vi "Sub_Online_FEA.vi"(8 "Bound Search":bool, 9 "Mode Count":i32=3 min=1 max=10 step=1, 10 "Eigenvalue Method":T2(ring), 11 "Experiment In":T1) -> (3 "Experiment Out":T1)   [LabVIEW 2021]
uses:
  <vilib>/Analysis/7linalg.llb/Eigenvalue and Vectors Output Option.ctl
  <vilib>/Analysis/baseanly.llb/Matrix Type of Inverse Matrix.ctl
  <vilib>/Analysis/7linalg.llb/Real Generalized Eigenvalues and Vectors.vi
  <vilib>/Analysis/7linalg.llb/Real Cholesky Factorization.vi
  <vilib>/Analysis/baseanly.llb/Full Cholesky Factorization.vi
  <vilib>/Analysis/baseanly.llb/Full Real Matrix Cholesky Factorization.vi
  <vilib>/Analysis/Matrix/Numeric/Conversions/Array To Matrix - RA2.vi
  <vilib>/Analysis/baseanly.llb/Real Inverse Matrix.vi
  <vilib>/Analysis/Matrix/Numeric/Multiply/Multiply - RM,RM.vi
  <vilib>/Analysis/7linalg.llb/Real Eigenvalues and Vectors.vi
  <vilib>/Analysis/Matrix/Numeric/Add/Add - RM,RM.vi
  <vilib>/Analysis/NI_AALPro.lvlib
  <vilib>/Analysis/Matrix/NI_Matrix.lvlib
  <vilib>/Analysis/NI_AALBase.lvlib
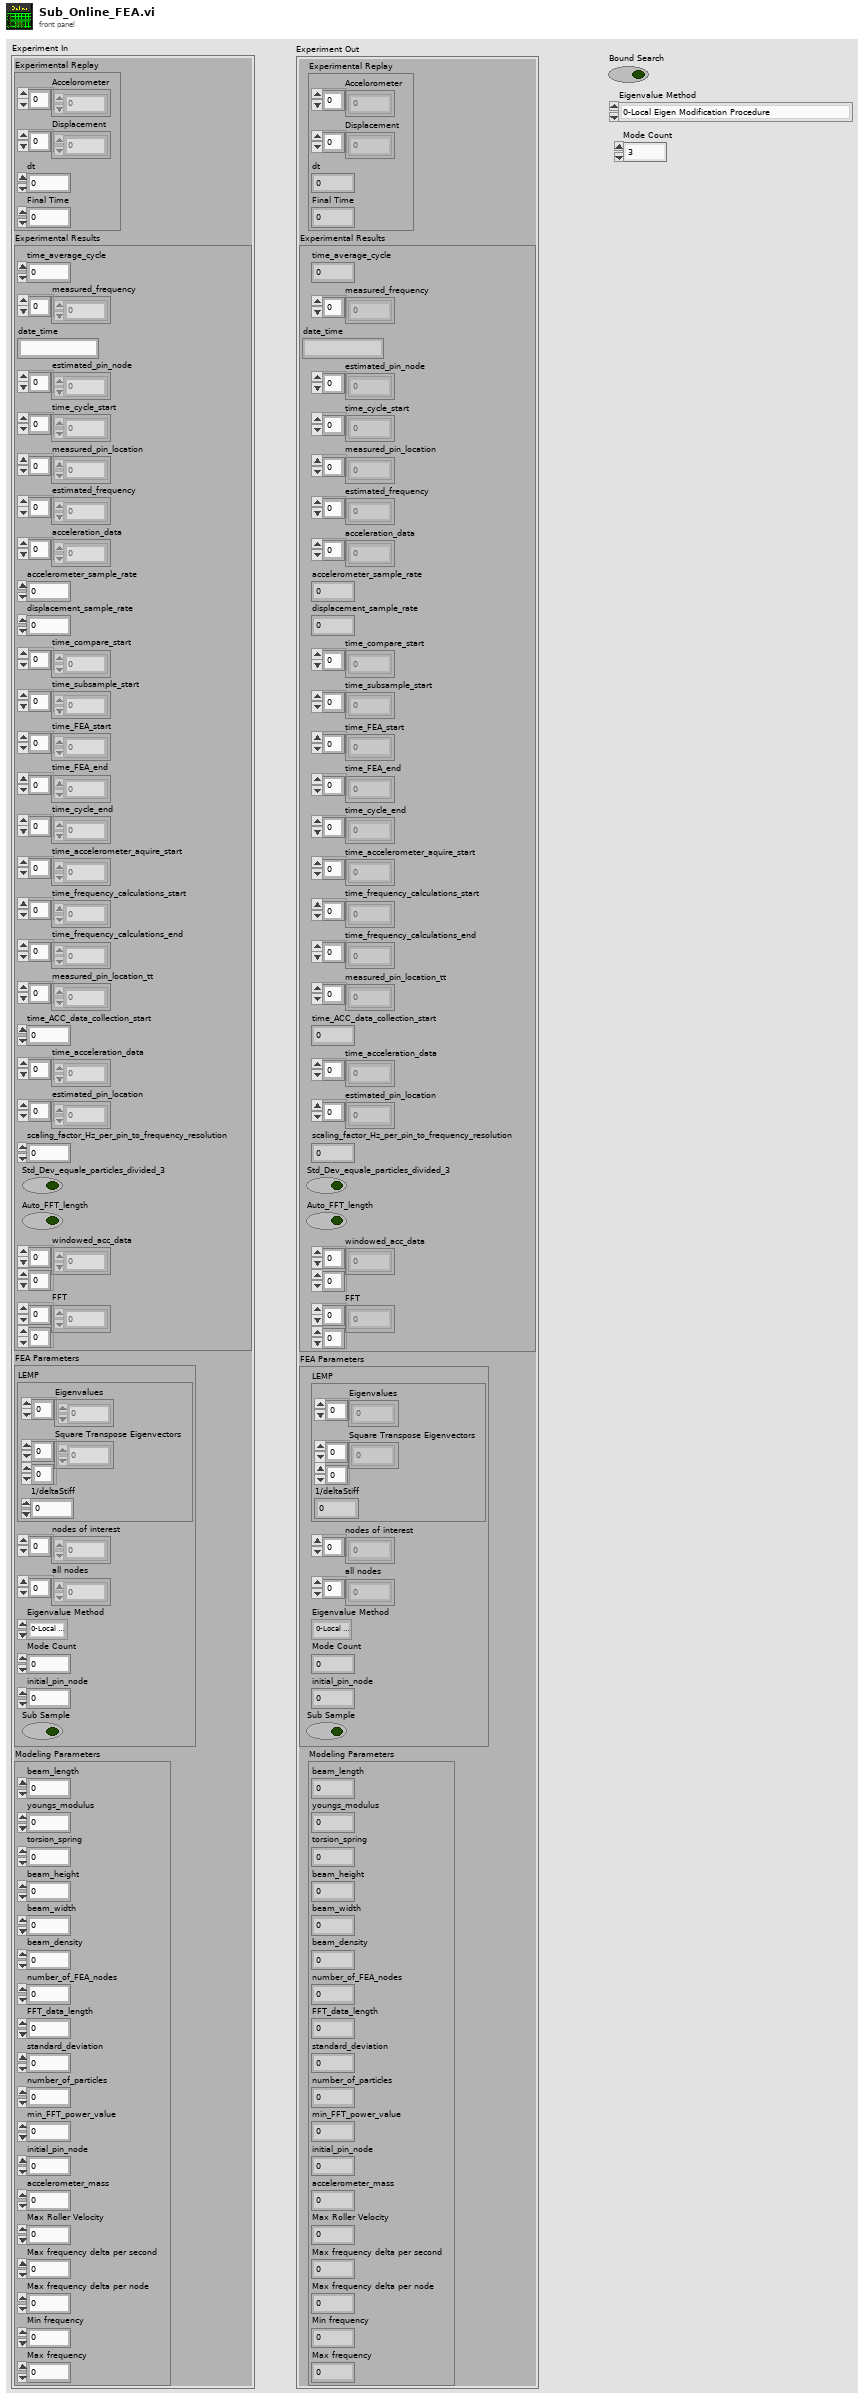
[diagram p1: front panel]
types:
  T1 = cluster{"Experimental Replay":cluster{"Accelorometer":dbl[], "Displacement":dbl[], "dt":dbl, "Final Time":dbl}, "Experimental Results":cluster{"time_average_cycle":dbl, "measured_frequency":dbl[], "date_time":string, "estimated_pin_node":i32[], "time_cycle_start":dbl[], "measured_pin_location":dbl[], "estimated_frequency":dbl[], "acceleration_data":dbl[], "accelerometer_sample_rate":dbl, "displacement_sample_rate":dbl, "time_compare_start":dbl[], "time_subsample_start":dbl[], "time_FEA_start":dbl[], "time_FEA_end":dbl[], "time_cycle_end":dbl[], "time_accelerometer_aquire_start":dbl[], "time_frequency_calculations_start":dbl[], "time_frequency_calculations_end":dbl[], "measured_pin_location_tt":dbl[], "time_ACC_data_collection_start":dbl, "time_acceleration_data":dbl[], "estimated_pin_location":dbl[], "scaling_factor_Hz_per_pin_to_frequency_resolution":dbl, "Std_Dev_equale_particles_divided_3":bool, "Auto_FFT_length":bool, "windowed_acc_data":dbl[][], "FFT":dbl[][]}, "FEA Parameters":cluster{"LEMP":cluster{"Eigenvalues":dbl[], "Square Transpose Eigenvectors":dbl[][], "1/deltaStiff":dbl}, "nodes of interest":i32[], "all nodes":i32[], "Eigenvalue Method":enum16{"0-Local Eigen Modification Procedure", "1-LabVIEW generalized eigenvalues", "2-LabVIEW M^-1K eigenvalues", "3-LabVIEW Cholesky Factorization", "4-Cholesky Factorization CPU SGL", "5-Cholesky Factorization CPU FXP", "6-Cholesky Factorization FPGA SGL", "7-Cholesky Factorization FPGA SGL SCL"}, "Mode Count":i32, "initial_pin_node":i32, "Sub Sample":bool}, "Modeling Parameters":cluster{"beam_length":dbl, "youngs_modulus":dbl, "torsion_spring":dbl, "beam_height":dbl, "beam_width":dbl, "beam_density":dbl, "number_of_FEA_nodes":i32, "FFT_data_length":i32, "standard_deviation":dbl, "number_of_particles":i32, "min_FFT_power_value":dbl, "initial_pin_node":i32, "accelerometer_mass":dbl, "Max Roller Velocity":dbl, "Max frequency delta per second":dbl, "Max frequency delta per node":dbl, "Min frequency":dbl, "Max frequency":dbl}}
  T2 = enum16{"0-Local Eigen Modification Procedure", "1-LabVIEW generalized eigenvalues", "2-LabVIEW M^-1K eigenvalues", "3-LabVIEW Cholesky Factorization", "4-Cholesky Factorization CPU SGL", "5-Cholesky Factorization CPU FXP", "6-Cholesky Factorization FPGA SGL", "7-Cholesky Factorization FPGA SGL SCL"}
  T3 = cluster{"LEMP":cluster{"Eigenvalues":dbl[], "Square Transpose Eigenvectors":dbl[][], "1/deltaStiff":dbl}, "nodes of interest":i32[], "all nodes":i32[], "Eigenvalue Method":enum16{"0-Local Eigen Modification Procedure", "1-LabVIEW generalized eigenvalues", "2-LabVIEW M^-1K eigenvalues", "3-LabVIEW Cholesky Factorization", "4-Cholesky Factorization CPU SGL", "5-Cholesky Factorization CPU FXP", "6-Cholesky Factorization FPGA SGL", "7-Cholesky Factorization FPGA SGL SCL"}, "Mode Count":i32, "initial_pin_node":i32, "Sub Sample":bool}
  T4 = cluster{"beam_length":dbl, "youngs_modulus":dbl, "torsion_spring":dbl, "beam_height":dbl, "beam_width":dbl, "beam_density":dbl, "number_of_FEA_nodes":i32, "FFT_data_length":i32, "standard_deviation":dbl, "number_of_particles":i32, "min_FFT_power_value":dbl, "initial_pin_node":i32, "accelerometer_mass":dbl, "Max Roller Velocity":dbl, "Max frequency delta per second":dbl, "Max frequency delta per node":dbl, "Min frequency":dbl, "Max frequency":dbl}
  T5 = cluster{"time_average_cycle":dbl, "measured_frequency":dbl[], "date_time":string, "estimated_pin_node":i32[], "time_cycle_start":dbl[], "measured_pin_location":dbl[], "estimated_frequency":dbl[], "acceleration_data":dbl[], "accelerometer_sample_rate":dbl, "displacement_sample_rate":dbl, "time_compare_start":dbl[], "time_subsample_start":dbl[], "time_FEA_start":dbl[], "time_FEA_end":dbl[], "time_cycle_end":dbl[], "time_accelerometer_aquire_start":dbl[], "time_frequency_calculations_start":dbl[], "time_frequency_calculations_end":dbl[], "measured_pin_location_tt":dbl[], "time_ACC_data_collection_start":dbl, "time_acceleration_data":dbl[], "estimated_pin_location":dbl[], "scaling_factor_Hz_per_pin_to_frequency_resolution":dbl, "Std_Dev_equale_particles_divided_3":bool, "Auto_FFT_length":bool, "windowed_acc_data":dbl[][], "FFT":dbl[][]}
  T6 = cluster{"Eigenvalues":dbl[], "Square Transpose Eigenvectors":dbl[][], "1/deltaStiff":dbl}
  T7 = typedef "NI_AALBase.lvlib/Matrix Type of Inverse Matrix.ctl" = enum32{"General", "Positive Definite", "Lower Triangular", "Upper Triangular"}
  T8 = typedef "NI_AALPro.lvlib/Eigenvalue and Vectors Output Option.ctl" = i32
  T9 = typedef "NI_Matrix.lvlib/RealMatrix.ctl" = dbl[][]
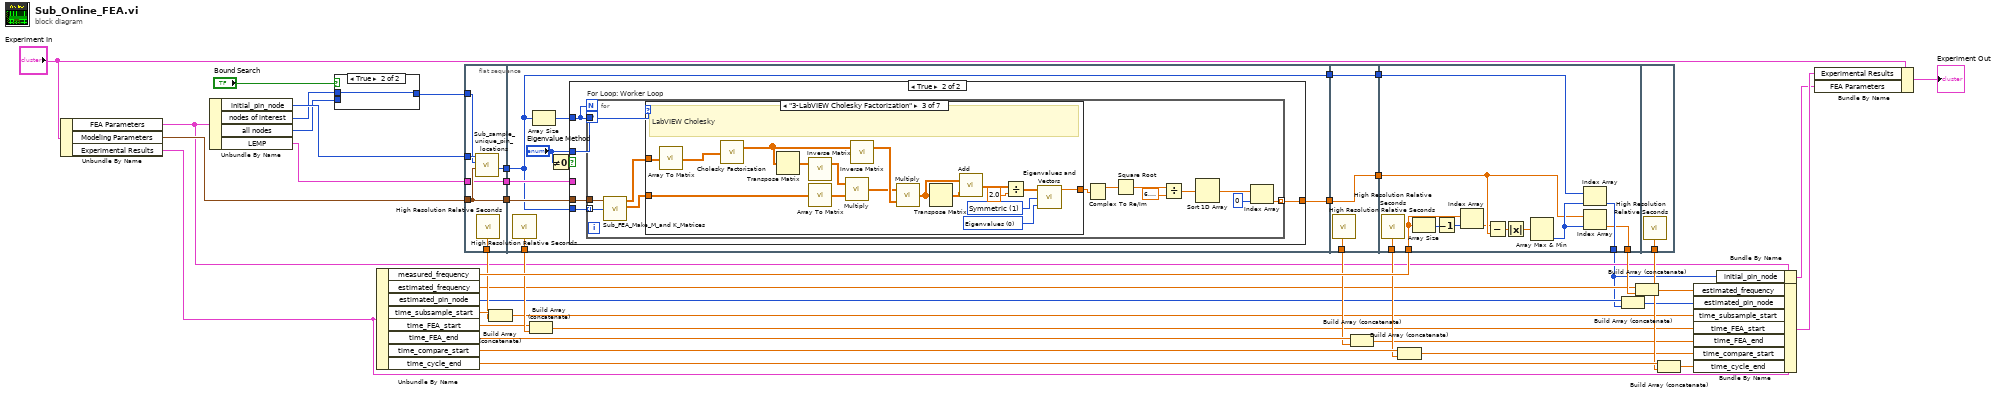
[diagram p0: block diagram]
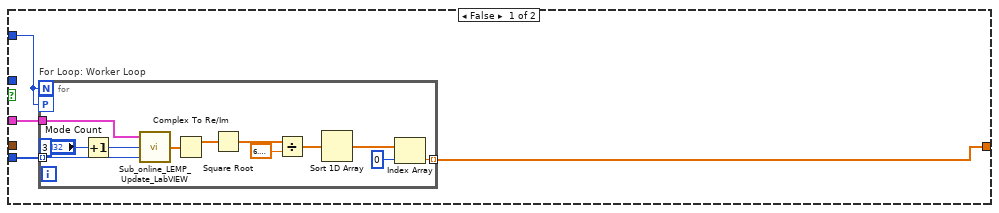
[diagram p3: hidden frame]
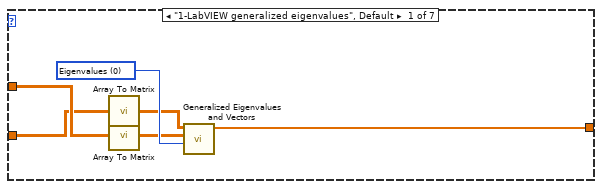
[diagram p4: hidden frame]
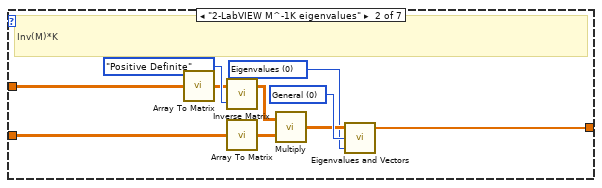
[diagram p5: hidden frame]
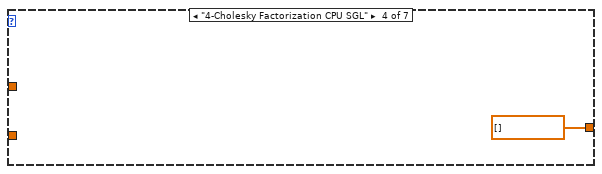
[diagram p6: hidden frame]
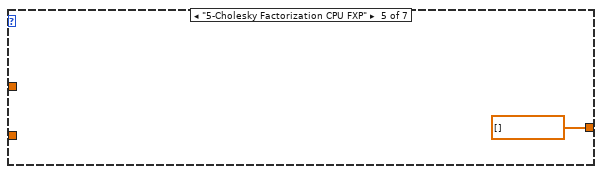
[diagram p7: hidden frame]
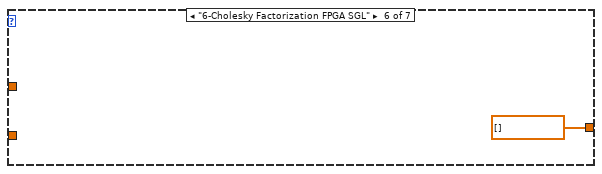
[diagram p8: hidden frame]
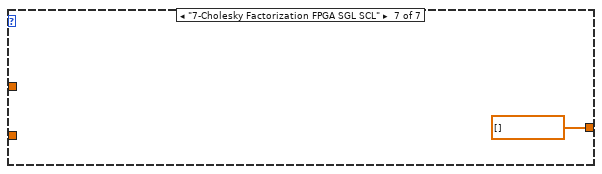
[diagram p9: hidden frame]
diagram:
  n1 = Unbundle By Name("Experiment In") -> ("FEA Parameters"=w3:T3, "Modeling Parameters"=w35:T4, "Experimental Results"=w14:T5)
  n2 = Unbundle By Name(w3) -> ("initial_pin_node"=w36:i32, "nodes of interest"=w34:i32[], "all nodes"=w33:i32[], "LEMP"=w32:T6)
  n3 = case shown="True" "Bound Search" {
    tunnel: w34 -> [_ w44]
    tunnel: w33 -> [w43 _]
    tunnel: [w43 w44] -> w37
    frame False {
    }
    frame True {
    }
  }
  n4 = Unbundle By Name(w14) -> ("measured_frequency"=w30:dbl[], "estimated_frequency"=w15:dbl[], "estimated_pin_node"=w16:i32[], "time_subsample_start"=w27:dbl[], "time_FEA_start"=w24:dbl[], "time_FEA_end"=w23:dbl[], "time_compare_start"=w21:dbl[], "time_cycle_end"=w19:dbl[])
  n5 = flat-sequence {
    tunnel: w35 -> [w48]
    tunnel: [w48] -> w42
    tunnel: w36 -> [w50]
    tunnel: [w49] -> w26
    tunnel: w32 -> [w47]
    tunnel: [w47] -> w41
    tunnel: [w46] -> w40
    tunnel: w37 -> [w45]
    tunnel: w42 -> [w57]
    tunnel: [w58] -> w39
    tunnel: [w56] -> w25
    tunnel: w41 -> [w53]
    tunnel: w40 -> [w51]
    tunnel: [w51] -> w28
    tunnel: w39 -> [w132]
    tunnel: [w132] -> w38
    tunnel: [w131] -> w22
    tunnel: [w130] -> w29
    tunnel: w28 -> [w130]
    tunnel: w38 -> [w142]
    tunnel: [w140] -> w20
    tunnel: w30 -> [w138]
    tunnel: w29 -> [w135]
    tunnel: [w134] -> w2
    tunnel: [w133] -> w17
    tunnel: [w145] -> w18
    frame #0 {
      n6 = call "Sub_sample_unique_pin_locations.vi"("Modeling Parameters"=w48, "FEA Nodes"=w45, "Initial Pin Location"=w50) -> ("Unique Samples"=w46:i32[])  [unwired: 6 in, 2 out]
      n7 = call <vilib>:"High Resolution Relative Seconds.vi"() -> ("relative seconds"=w49:dbl)
    }
    frame #1 {
      n8 = call <vilib>:"High Resolution Relative Seconds.vi"() -> ("relative seconds"=w56:dbl)
      n9 = Array Size(array=w51) -> (size(s)=w52:i32)
      n10 = Not Equal To 0?(x="Eigenvalue Method") -> (x != 0?=w55:bool)
      n11 = case shown="True" w55 {
        tunnel: w51 -> [w61 w79]
        tunnel: [w60 w78] -> w58
        tunnel: w57 -> [_ w77]
        tunnel: w52 -> [w62 w76]
        tunnel: "Eigenvalue Method" -> [_ w75]
        tunnel: w53 -> [w59 _]
        frame False {
          n12 = for "For Loop: Worker Loop" {
            N: w62 -> [_]
            workers-P: w62 -> [_]
            tunnel: w61 -> [w64] mode=indexing
            tunnel: [w68] -> w60 mode=indexing
            tunnel: w59 -> [w63]
            (unwired) 3 ("Mode Count")
            n13 = Increment(x="Mode Count") -> (x+1=w65:i32)
            n14 = call "Sub_online_LEMP_Update_LabVIEW.vi"("Effected DOF"=w64, "Mode count"=w65, "LEMP"=w63) -> ("Updated Eigenvalues"=w67:dbl[])
            n15 = Complex To Re/Im ("Complex To Cartesian.vi")(x + iy=w67) -> (x=w74:dbl[])  [unwired: 1 out]
            n16 = Square Root ("Square Root.vi")(x=w74) -> (sqrt(x)=w73:dbl[])
            n17 = Divide(x=w73, y=6.283185307179586) -> (x/y=w69:dbl[])
            n18 = Sort 1D Array(array=w69) -> (sorted array=w71:dbl[])
            n19 = Index Array(array=w71, index=0) -> (element=w68:dbl)
          }
        }
        frame True {
          n20 = for "For Loop: Worker Loop" {
            N: w76 -> [_]
            tunnel: [w87] -> w78 mode=indexing
            tunnel: w79 -> [w84] mode=indexing
            tunnel: w77 -> [w80]
            workers-P: w76 -> [_]
            tunnel: w75 -> [w81]
            n21 = call "Sub_FEA_Make_M_and K_Matrices.vi"("Pin Location"=w84, "Modeling Parameters"=w80) -> ("K Matrix"=w83:dbl[][], "M Matrix"=w82:dbl[][])  [unwired: 8 in]
            n22 = case shown="\"3-LabVIEW Cholesky Factorization\"" w81 {
              tunnel: w82 -> [w96 w102 w110 _ _ _ _]
              tunnel: w83 -> [w95 w100 w112 _ _ _ _]
              tunnel: [w97 w105 w113 cdb[] [] ("Eigenvalues") cdb[] [] ("Eigenvalues") cdb[] [] ("Eigenvalues") cdb[] [] ("Eigenvalues")] -> w85
              frame "1-LabVIEW generalized eigenvalues", Default {
                w98 = T8 0 items=["Eigenvalues", "Eigenvalues & Vectors"] ("output option")
                n23 = call-poly <vilib>:"Array To Matrix.vi"("Real 2D Array"=w95) -> ("Real Matrix"=w94:T9)
                n24 = call-poly <vilib>:"Array To Matrix.vi"("Real 2D Array"=w96) -> ("Real Matrix"=w93:T9)
                n25 = call-poly <vilib>:"Generalized Eigenvalues and Vectors.vi"("output option"=w98, "B"=w93, "A"=w94) -> ("Eigenvalues"=w97:cdb[])  [unwired: 3 in, 2 out]
              }
              frame "2-LabVIEW M^-1K eigenvalues" {
                w104 = T8 0 items=["Eigenvalues", "Eigenvalues & Vectors"] ("output option")
                w107 = 0 items=["General", "Symmetric"] ("matrix type")
                # "Inv(M)*K"
                n26 = call-poly <vilib>:"Array To Matrix.vi"("Real 2D Array"=w102) -> ("Real Matrix"=w101:T9)
                n27 = call-poly <vilib>:"Inverse Matrix.vi"("matrix type"=Matrix_Type_of_Inverse_Matrix."Positive Definite", "Input Matrix"=w101) -> ("Inverse Matrix"=w108:T9)  [unwired: 1 out]
                n28 = call-poly <vilib>:"Array To Matrix.vi"("Real 2D Array"=w100) -> ("Real Matrix"=w99:T9)
                n29 = call-poly <vilib>:"Multiply.vi"("Real Matrix B"=w99, "Real Matrix A"=w108) -> ("A * B"=w106:T9)
                n30 = call-poly <vilib>:"Eigenvalues and Vectors.vi"("output option"=w104, "matrix type"=w107, "Input Matrix"=w106) -> ("Eigenvalues"=w105:cdb[])  [unwired: 2 out]
              }
              frame "3-LabVIEW Cholesky Factorization" {
                w115 = T8 0 items=["Eigenvalues", "Eigenvalues & Vectors"] ("output option")
                w116 = 1 items=["General", "Symmetric"] ("matrix type")
                # "LabVIEW Cholesky"
                n31 = call-poly <vilib>:"Array To Matrix.vi"("Real 2D Array"=w110) -> ("Real Matrix"=w109:T9)
                n32 = call-poly <vilib>:"Cholesky Factorization.vi"("A"=w109) -> ("Cholesky"=w124:T9)  [unwired: 1 out]
                n33 = Transpose Matrix(1:w124) -> (0:w125:T9)
                n34 = call-poly <vilib>:"Inverse Matrix.vi"("Input Matrix"=w125) -> ("Inverse Matrix"=w123:T9)  [unwired: 1 in, 1 out]
                n35 = call-poly <vilib>:"Array To Matrix.vi"("Real 2D Array"=w112) -> ("Real Matrix"=w111:T9)
                n36 = call-poly <vilib>:"Multiply.vi"("Real Matrix B"=w111, "Real Matrix A"=w123) -> ("A * B"=w121:T9)
                n37 = call-poly <vilib>:"Inverse Matrix.vi"("Input Matrix"=w124) -> ("Inverse Matrix"=w122:T9)  [unwired: 1 in, 1 out]
                n38 = call-poly <vilib>:"Multiply.vi"("Real Matrix B"=w122, "Real Matrix A"=w121) -> ("A * B"=w120:T9)
                n39 = Transpose Matrix(1:w120) -> (0:w119:T9)
                n40 = call-poly <vilib>:"Add.vi"("Real Matrix B"=w119, "Real Matrix A"=w120) -> ("A + B"=w117:T9)
                n41 = Divide(x=w117, y=2.0) -> (x/y=w114:T9)
                n42 = call-poly <vilib>:"Eigenvalues and Vectors.vi"("output option"=w115, "matrix type"=w116, "Input Matrix"=w114) -> ("Eigenvalues"=w113:cdb[])  [unwired: 2 out]
              }
              frame "4-Cholesky Factorization CPU SGL" {
              }
              frame "5-Cholesky Factorization CPU FXP" {
              }
              frame "6-Cholesky Factorization FPGA SGL" {
              }
              frame "7-Cholesky Factorization FPGA SGL SCL" {
              }
            }
            n43 = Complex To Re/Im ("Complex To Cartesian.vi")(x + iy=w85) -> (x=w92:dbl[])  [unwired: 1 out]
            n44 = Square Root ("Square Root.vi")(x=w92) -> (sqrt(x)=w91:dbl[])
            n45 = Divide(x=w91, y=6.283185307179586) -> (x/y=w86:dbl[])
            n46 = Sort 1D Array(array=w86) -> (sorted array=w89:dbl[])
            n47 = Index Array(array=w89, index=0) -> (element=w87:dbl)
          }
        }
      }
    }
    frame #2 {
      n48 = call <vilib>:"High Resolution Relative Seconds.vi"() -> ("relative seconds"=w131:dbl)
    }
    frame #3 {
      n49 = call <vilib>:"High Resolution Relative Seconds.vi"() -> ("relative seconds"=w140:dbl)
      n50 = Array Size(array=w138) -> (size(s)=w136:i32)
      n51 = Decrement(x=w136) -> (x-1=w137:i32)
      n52 = Index Array(array=w138, index=w137) -> (element=w139:dbl)
      n53 = Subtract(x=w139, y=w142) -> (x-y=w144:dbl[])
      n54 = Absolute Value(x=w144) -> (abs(x)=w141:dbl[])
      n55 = Array Max & Min(array=w141) -> (min index (indices)=w143:i32)  [unwired: 3 out]
      n56 = Index Array(array=w135, index=w143) -> (element=w134:i32)
      n57 = Index Array(array=w142, index=w143) -> (element=w133:dbl)
    }
    frame #4 {
      n58 = call <vilib>:"High Resolution Relative Seconds.vi"() -> ("relative seconds"=w145:dbl)
    }
  }
  n59 = Build Array (concatenate)(w27, w26) -> (w7:dbl[])
  n60 = Build Array (concatenate)(w24, w25) -> (w8:dbl[])
  n61 = Build Array (concatenate)(w23, w22) -> (w11:dbl[])
  n62 = Build Array (concatenate)(w21, w20) -> (w12:dbl[])
  n63 = Build Array (concatenate)(w16, w2) -> (w10:i32[])
  n64 = Build Array (concatenate)(w15, w17) -> (w9:dbl[])
  n65 = Build Array (concatenate)(w19, w18) -> (w13:dbl[])
  n66 = Bundle By Name(cluster=w14, "estimated_frequency"=w9, "estimated_pin_node"=w10, "time_subsample_start"=w7, "time_FEA_start"=w8, "time_FEA_end"=w11, "time_compare_start"=w12, "time_cycle_end"=w13) -> (w4:T5)
  n67 = Bundle By Name(cluster=w3, "initial_pin_node"=w2) -> (w1:T3)
  n68 = Bundle By Name(cluster="Experiment In", "Experimental Results"=w4, "FEA Parameters"=w1) -> (→"Experiment Out":T1)
